vi "Sideways Calculate Particle Scores.vi"(6 "Expected Aspect Ratio":dbl=1.6 format="%#_13g", 7 "Pixel Value":i32=1, 8 "Limit Tests?":bool=TRUE, 9 "Aspect Fudge Factor":dbl=1.0, 10 "Sorted Data":dbl[][](array[numeric]), 11 "Image in":T2) -> (3 "Scores":T1(array[cluster]))   [LabVIEW 2015]
doc: "Calculate scores based on the particle measurements. Calculated scores are for aspect ratio, area to convex hull area, masking, and moment of inertia. These scores range between 0 and 100 and can be used to categorize particles as targets and non-targets. The fudge factor compensates for camera modes that do not give square pixels."
uses:
  <vilib>/vision/Image Controls.llb/IMAQ Image.ctl
  <vilib>/vision/NI_Vision_Development_Module.lvlib
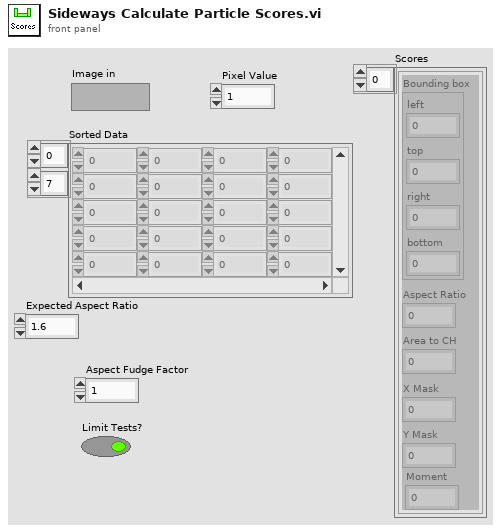
[diagram p1: front panel]
types:
  T1 = cluster{"Bounding box":cluster{"left":dbl, "top":dbl, "right":dbl, "bottom":dbl}, "Aspect Ratio":dbl, "Area to CH":dbl, "X Mask":dbl, "Y Mask":dbl, "Moment":dbl}[]
  T2 = typedef "IMAQ Image.ctl" = refnum<image>
  T3 = cluster{"[0]":dbl, "[1]":dbl, "[2]":dbl, "[3]":dbl}
  T4 = cluster{cluster{"[0]":dbl, "[1]":dbl, "[2]":dbl, "[3]":dbl}, "Aspect Ratio Score":dbl, "Score":dbl, "X Score":dbl, "Y Score":dbl, "Score":dbl}
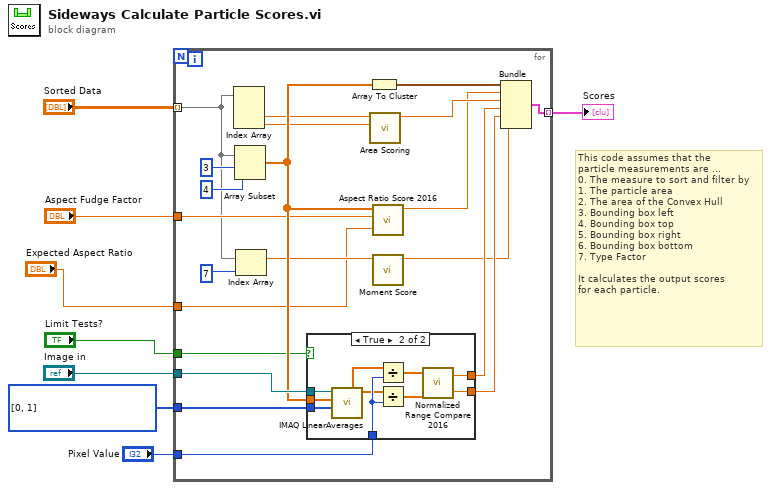
[diagram p0: block diagram]
diagram:
  w6 = i32[] [0, 1] items=["X Axis Averages", "Y Axis Averages", "X + Y Axis Averages", "X - Y Axis Averages"] ("Averages")
  # "This code assumes that the\nparticle measurements are ...\n0. The measure to sort and filter by\n1. The particle area\n2. The area of the Convex Hull\n3. Bounding box left\n4. Bounding box top\n5. Bounding box right\n6. Bounding box bottom\n7. Type Factor\n\nIt calculates the output scores\nfor each particle."
  n1 = for {
    tunnel: "Image in" -> [w25]
    tunnel: "Sorted Data" -> [w13] mode=indexing
    tunnel: [w27] -> w7 mode=indexing
    tunnel: w6 -> [w20]
    tunnel: "Pixel Value" -> [w18]
    tunnel: "Aspect Fudge Factor" -> [w15]
    tunnel: "Limit Tests?" -> [w14]
    tunnel: "Expected Aspect Ratio" -> [w9]
    n2 = Index Array(array=w13) -> (element #2=w17:dbl, element #3=w16:dbl)  [unwired: 3 in, 1 out]
    n3 = Array Subset(array=w13, index=3, length=4) -> (w19:dbl[])
    n4 = Index Array(array=w13, index=7 ("length")) -> (element=w11:dbl)
    n5 = case shown="True" w14 {
      tunnel: w25 -> [_ w39]
      tunnel: [_ w38] -> w22
      tunnel: [_ w37] -> w21
      tunnel: w20 -> [_ w36]
      tunnel: w19 -> [_ w35]
      tunnel: w18 -> [_ w34]
      frame False {
      }
      frame True {
        n6 = call "IMAQ LinearAverages"("Averages"=w36, "Optional Rectangle"=w35, "Image Src"=w39) -> ("Y Axis Averages"=w32:sgl[], "X Axis Averages"=w33:sgl[])  [unwired: 4 in, 3 out]
        n7 = Divide(x=w33, y=w34) -> (x/y=w31:sgl[])
        n8 = Divide(x=w32, y=w34) -> (x/y=w30:sgl[])
        n9 = call "Normalized Range Compare 2016.vi"("Y Averages"=w30, "X Averages"=w31) -> ("Y Score"=w37:dbl, "X Score"=w38:dbl)
      }
    }
    n10 = Array To Cluster(array=w19) -> (cluster=w24:T3)
    n11 = call "Area Scoring.vi"("Convex Hull Area"=w16, "Area"=w17) -> ("Score"=w26:dbl)  [unwired: 9 in]
    n12 = call "Aspect Ratio Score 2016.vi"("Expected Aspect Ratio"=w9, "Aspect Fudge Factor"=w15, "Rectangle Array ltrb"=w19) -> ("Aspect Ratio Score"=w23:dbl)  [unwired: 8 in]
    n13 = call "Moment Score.vi"("Moment Factor"=w11) -> ("Score"=w10:dbl)  [unwired: 10 in]
    n14 = Bundle(w24, "Aspect Ratio Score"=w23, "Score"=w26, "X Score"=w22, "Y Score"=w21, "Score"=w10) -> (w27:T4)  [unwired: 1 in]
  }
  "Scores" <- w7
